vi "Config aNETka.vi"() -> (0 "Continue? (T=yes)":bool=TRUE, 1 "1D ANN config":i32[](array[numeric])=[2, 5, 1])   [LabVIEW 2010]
panel:
  out "Wait...":string="Wait..."
  out "Map of the neural network (node configuration)":cluster{dbl[], dbl[]}[](graph)=[{[2.0, 3.0], [5.5, 3.5]}, {[2.0, 3.0], [4.5, 3.5]}, {[2.0, 3.0], [3.5, 3.5]}, {[2.0, 3.0], [2.5, 3.5]}, {[2.0, 3.0], [1.5, 3.5]}, {[1.0, 2.0], [4.0, 1.5]}, {[1.0, 2.0], [4.0, 2.5]}, {[1.0, 2.0], [4.0, 3.5]}, {[1.0, 2.0], [4.0, 4.5]}, {[1.0, 2.0], [4.0, 5.5]}, {[1.0, 2.0], [3.0, 1.5]}, {[1.0, 2.0], [3.0, 2.5]}, {[1.0, 2.0], [3.0, 3.5]}, {[1.0, 2.0], [3.0, 4.5]}, {[1.0, 2.0], [3.0, 5.5]}]
  in  "Exit":bool
  in  "OK":bool
  in  "1D ANN config":i32[](array[numeric])=[2, 5, 1] caption="Configuration\nof max. 8 layer:\nFirst=inputs,\nmiddle=hidden,\nlast=outputs \n(first zero ends\nconfiguration)" min=0 max=100 step=1
  # "Please configure aNETka..."
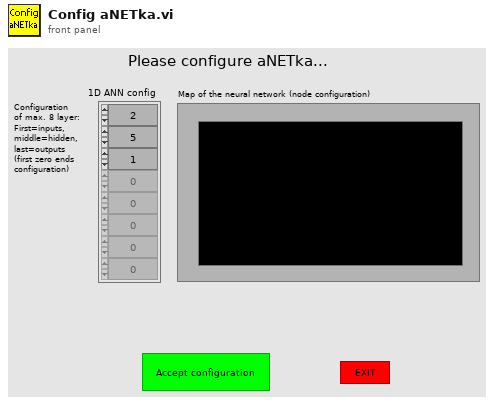
[diagram p1: front panel]
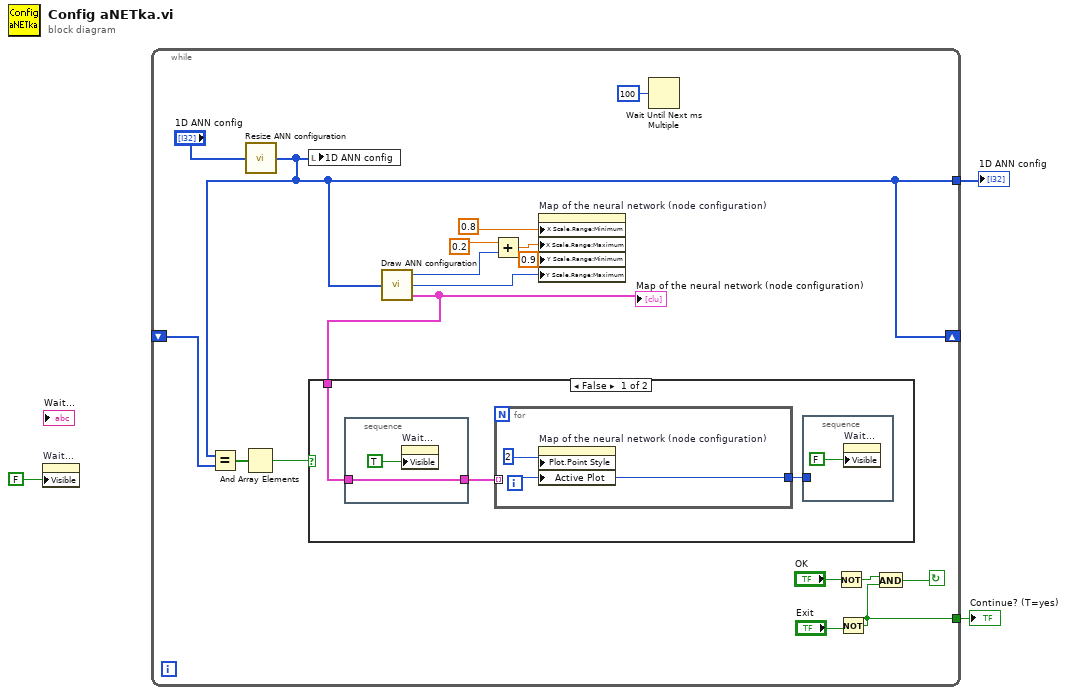
[diagram p0: block diagram]
diagram:
  n1 = property on="Wait..." class="Str"("Visible"=FALSE ("Write Attribute")) -> ()  [unwired: 2 in, 2 out]
  n2 = while {
    tunnel: [w5] -> w1
    shift-left: _ -> [w12]
    shift-right: [w8] -> _
    tunnel: [w8] -> w2
    stop <- w6 continue-if-true
    n3 = call "Resize ANN configuration.vi"("Configuration\nof layers"="1D ANN config") -> ("Resized configuration\n(if necessary)"=w8:i32[])
    n4 = Equal?(x=w8, y=w12) -> (x = y?=w11:bool[])
    n5 = And Array Elements(Boolean array=w11) -> (logical AND=w10:bool)
    n6 = local write "1D ANN config"(w8) -> ()
    n7 = call "Draw ANN configuration.vi"("Array"=w8) -> ("Xmax"=w19:i8, "Ymax"=w16:i16, "Map of the neural network (node configuration)"=w13:cluster{dbl[], dbl[]}[])
    "Map of the neural network (node configuration)" <- w13
    n8 = case shown="False" w10 {
      tunnel: w13 -> [w23 _]
      frame False {
        n9 = stacked-sequence {
          tunnel: w23 -> [w26]
          tunnel: [w26] -> w24
          frame #0 {
            n10 = property on="Wait..." class="Str"("Visible"=TRUE ("Write Attribute")) -> ()  [unwired: 2 in, 2 out]
          }
        }
        n11 = for {
          tunnel: [w29] -> w22
          tunnel: w24 -> [_] mode=indexing
          i -> [w29]
          n12 = property on="Map of the neural network (node configuration)" class="XYGraph (strict)"("Plot.Point Style"=u8 2 ("Write Attribute"), "Active Plot"=w29) -> ()  [unwired: 2 in, 2 out]
        }
        n13 = stacked-sequence {
          tunnel: w22 -> [_]
          frame #0 {
            n14 = property on="Wait..." class="Str"("Visible"=FALSE ("Write Attribute")) -> ()  [unwired: 2 in, 2 out]
          }
        }
      }
      frame True {
      }
    }
    n15 = Add(x=0.2, y=w19) -> (x+y=w17:dbl)
    n16 = property on="Map of the neural network (node configuration)" class="XYGraph (strict)"("X Scale.Range:Minimum"=0.8, "X Scale.Range:Maximum"=w17, "Y Scale.Range:Minimum"=0.9, "Y Scale.Range:Maximum"=w16) -> ()  [unwired: 2 in, 2 out]
    n17 = Wait Until Next ms Multiple(millisecond multiple=u32 100) -> ()  [unwired: 1 out]
    n18 = Not(x="OK") -> (.not. x?=w20:bool)
    n19 = Not(x="Exit") -> (.not. x?=w5:bool)
    n20 = And(x=w20, y=w5) -> (x .and. y?=w6:bool)
  }
  "1D ANN config" <- w2
  "Continue? (T=yes)" <- w1
